vi "Parse Time.vi"(8 "error in (no error)":errorcluster, 11 "data":string) -> (0 "error out":errorcluster, 3 "Time Stamp":timestamp)   [LabVIEW 2018]
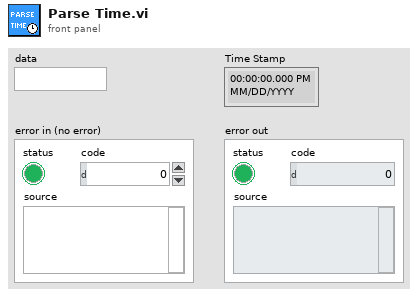
[diagram p1: front panel]
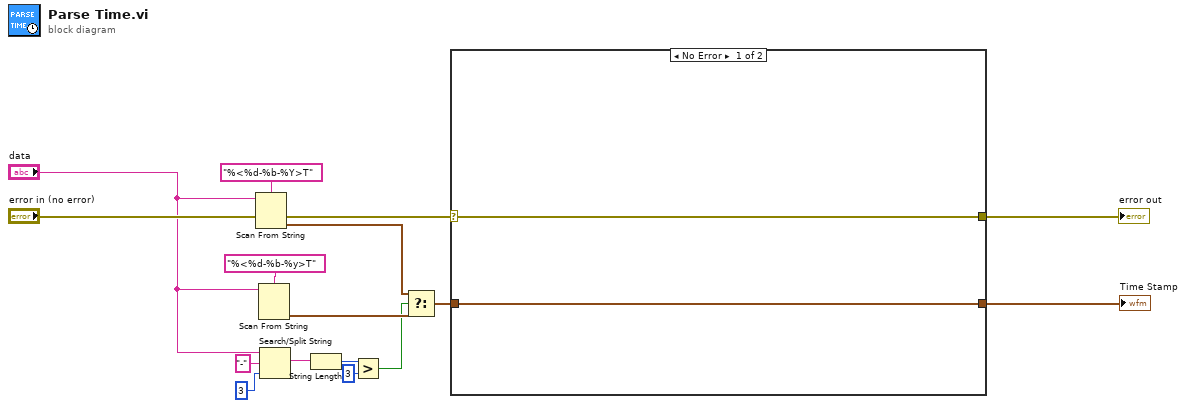
[diagram p0: block diagram]
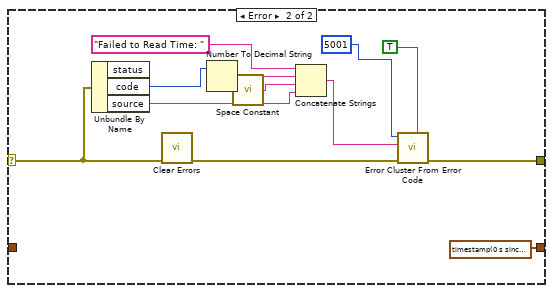
[diagram p2: hidden frame]
diagram:
  n1 = Scan From String(format string="%<%d-%b-%Y>T", input string="data", error in="error in (no error)") -> (error out=w15:errorcluster, output 1=w9:timestamp)  [unwired: 2 in, 2 out]
  n2 = Scan From String(format string="%<%d-%b-%y>T", input string="data") -> (output 1=w8:timestamp)  [unwired: 3 in, 3 out]
  n3 = Search/Split String(string="data", search string/char (-)="-", offset (0)=3) -> (match + rest of string=w4:string)  [unwired: 2 out]
  n4 = String Length(string=w4) -> (length=w3:i32)
  n5 = Greater?(x=w3, y=3) -> (0:w1:bool)
  n6 = Select(t=w9, s=w1, f=w8) -> (s? t:f=w10:timestamp)
  n7 = case shown="No Error" w15 {
    selector: w15 -> [w18 w26]
    tunnel: [w18 w28] -> w14
    tunnel: [w17 timestamp(0 s since 1904-01-01)] -> w13
    tunnel: w10 -> [w17 _]
    frame No Error {
    }
    frame Error {
      n8 = Unbundle By Name(w26) -> ("code"=w23:i32, "source"=w22:string)  [unwired: 1 out]
      n9 = call <vilib>:"Clear Errors.vi"("error in (no error)"=w26) -> ("error out"=w27:errorcluster)  [unwired: 5 in, 1 out]
      n10 = Number To Decimal String(number=w23) -> (decimal integer string=w20:string)  [unwired: 1 in]
      n11 = call <vilib>:"Space Constant.vi"() -> ("String"=w21:string)
      n12 = Concatenate Strings("Failed to Read Time: " ("error message (\"\")"), w20, w21, w22) -> (w19:string)
      n13 = call <vilib>:"Error Cluster From Error Code.vi"("is warning? (False)"=TRUE, "error in (no error)"=w27, "error message (\"\")"=w19, "error code (0)"=5001) -> ("error out"=w28:errorcluster)  [unwired: 5 in]
    }
  }
  "error out" <- w14
  "Time Stamp" <- w13
